vi "ClearSubPanel.vi"(8 "error in":errorcluster, 10 "user event ref":T1, 11 "sub panel ref in":refnum<vi>) -> (0 "error out":errorcluster, 3 "sub panel ref out":refnum<vi>)   [LabVIEW 2013, in "NISE_CEF_TreeControl.lvlib"]
uses:
  NISE_CEF_TreeControl.lvlib
  Node/UserEventRef.ctl
  Controls/EventCluster.ctl
  Node/NISE_CEF_Node.lvclass
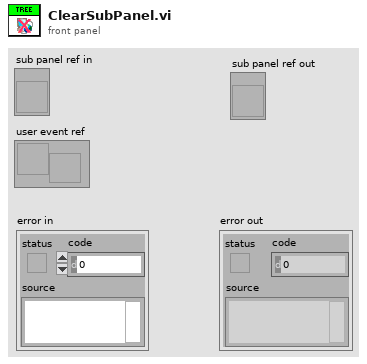
[diagram p1: front panel]
types:
  T1 = typedef "NISE_CEF_Node.lvclass/UserEventRef.ctl" = refnum<user-event>
  T2 = typedef "NISE_CEF_TreeControl.lvlib/EventCluster.ctl" = cluster{"command":string, "data":string}
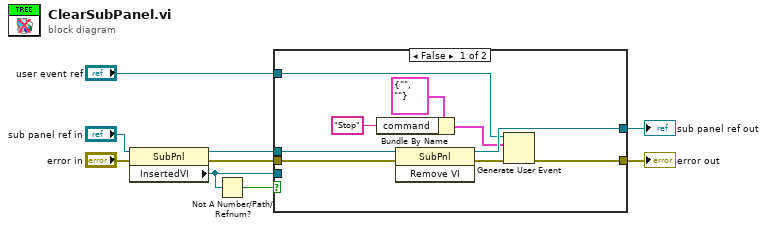
[diagram p0: block diagram]
diagram:
  n1 = property class="SubPnl"(reference="sub panel ref in", error in="error in") -> (reference out=w9:refnum<vi>, error out=w7:errorcluster, "InsertedVI"=w5:refnum<vi>)
  n2 = Not A Number/Path/Refnum?(number/path/refnum=w5) -> (NaN/Path/Refnum?=w8:bool)
  n3 = case shown="False" w8 {
    tunnel: [w13 w20] -> w2
    tunnel: w5 -> [_ _]
    tunnel: w9 -> [w18 w19]
    tunnel: w7 -> [w15 w20]
    tunnel: [w17 w19] -> w3
    tunnel: "user event ref" -> [w16 _]
    frame False {
      n4 = Bundle By Name(cluster=T2 {"command"="", "data"=""} ("event data"), "command"="Stop") -> (w11:T2)
      n5 = invoke class="SubPnl" method="Remove VI"(reference=w18, error in=w15) -> (reference out=w17:refnum<vi>, error out=w14:errorcluster)  [unwired: 1 in, 1 out]
      n6 = Generate User Event(user event=w16, event data cluster=w11, error in=w14) -> (error out=w13:errorcluster)  [unwired: 1 in, 1 out]
    }
    frame True {
      # "Reference is not valid if there is no VI"
    }
  }
  "error out" <- w2
  "sub panel ref out" <- w3
